vi "LEDS.vi"(7 "Action":T1, 8 "error in":errorcluster, 10 "On/Off":bool) -> (0 "error out":errorcluster)   [LabVIEW 2013]
uses:
  LEDSaction.ctl
  <vilib>/Rock Robotics/SystemInterfaces/DIO/FPGA_DIOChannel.ctl
  <vilib>/Rock Robotics/SystemInterfaces/Typedef/FPGA_TypedefDigitalModule.ctl
panel:
  out "PressureHigh":bool
  out "PressureLow":bool
  out "Shoot":bool
  out "Shift":bool
  out "Hot":bool
  out "NotHot":bool
  out "10 Seconds":bool
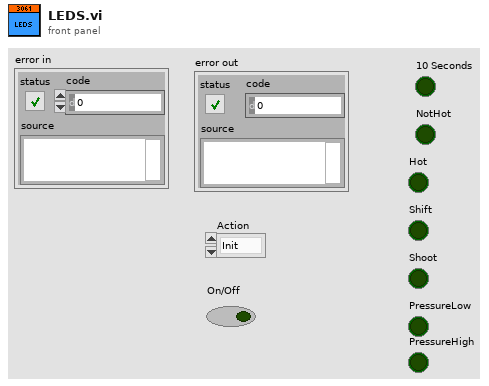
[diagram p1: front panel]
types:
  T1 = typedef "LEDSaction.ctl" = enum16{"Init", "10SecondsLeft", "LimitDown", "LimitUp", "CollectDown", "CollectUp", "NotHot", "Hot", "Shift", "RollBack", "RollFwd", "Shoot", "Distance Low", "DistanceHigh", "PressureLow", "PressureHigh"}
  T2 = typedef "FPGA_DIOChannel.ctl" = enum8{"DIO 1", "DIO 2", "DIO 3", "DIO 4", "DIO 5", "DIO 6", "DIO 7", "DIO 8", "DIO 9", "DIO 10", "DIO 11", "DIO 12", "DIO 13", "DIO 14", "Invalid"}
  T3 = typedef "FPGA_TypedefDigitalModule.ctl" = enum16{"Digital Module 1", "Digital Module 2"}
  T4 = typedef "WPI_DigitalOutputDevRef.ctl" = cluster{"Digital Module":T3, "DIO Channel":T2, "DevStatus":errorcluster}
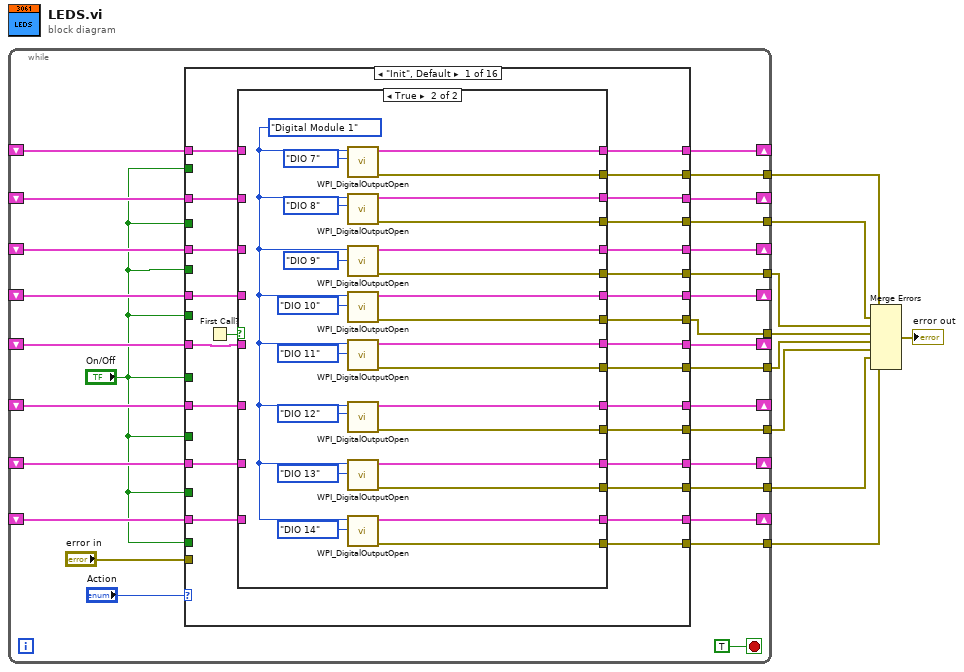
[diagram p0: block diagram]
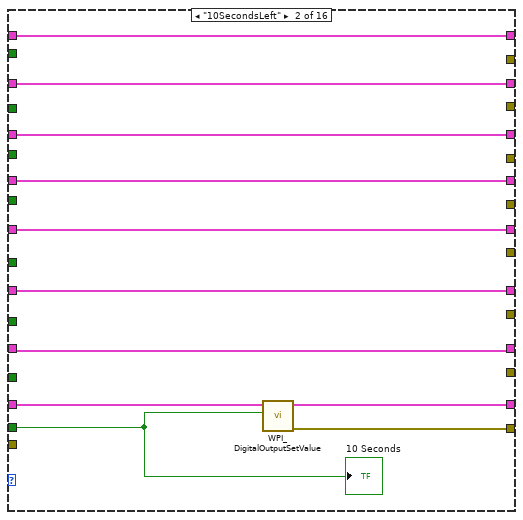
[diagram p3: hidden frame]
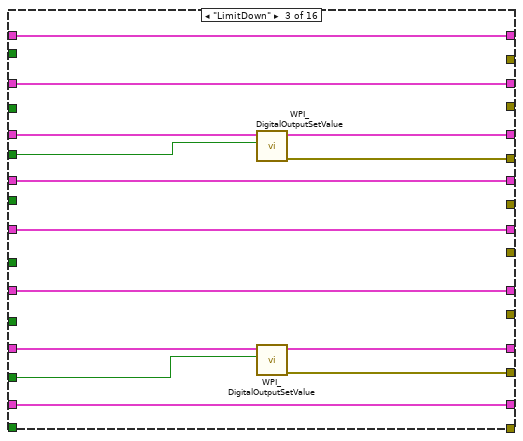
[diagram p4: hidden frame]
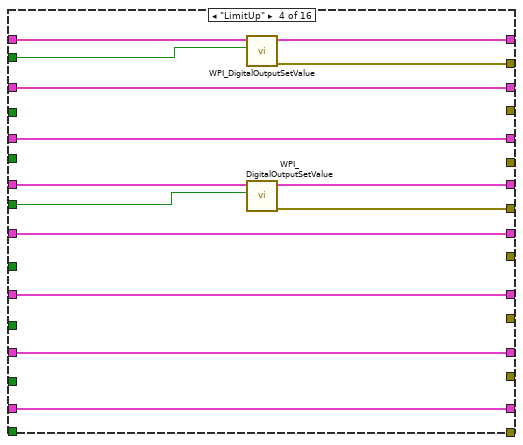
[diagram p5: hidden frame]
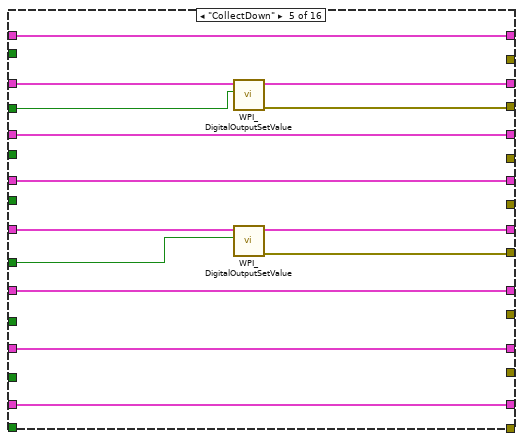
[diagram p6: hidden frame]
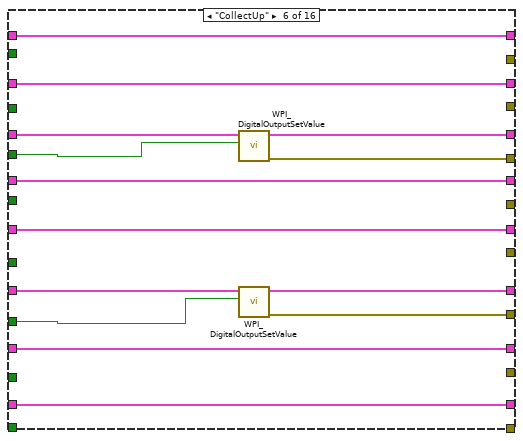
[diagram p7: hidden frame]
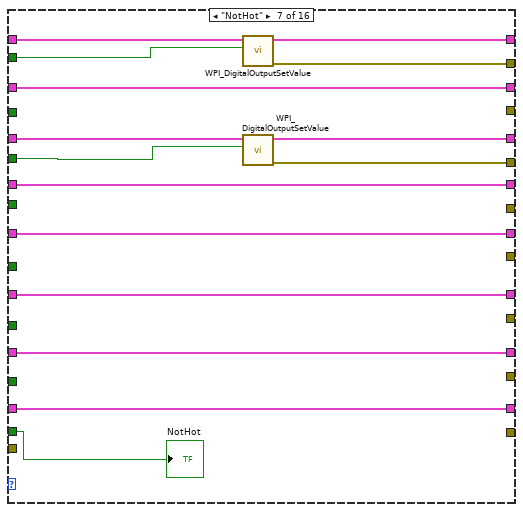
[diagram p8: hidden frame]
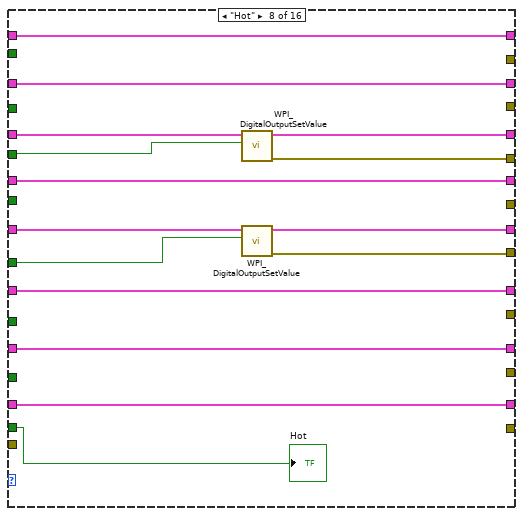
[diagram p9: hidden frame]
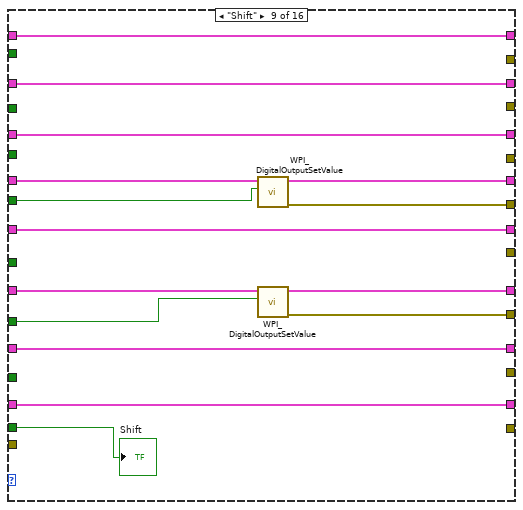
[diagram p10: hidden frame]
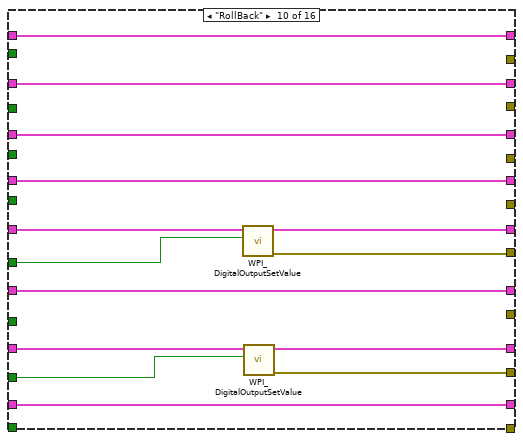
[diagram p11: hidden frame]
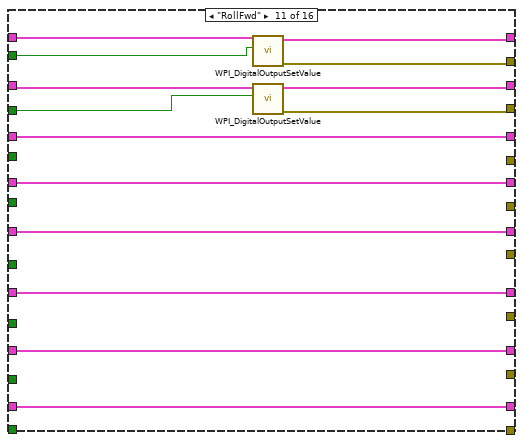
[diagram p12: hidden frame]
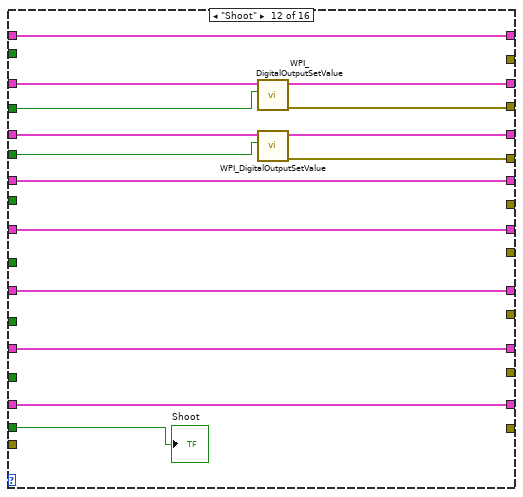
[diagram p13: hidden frame]
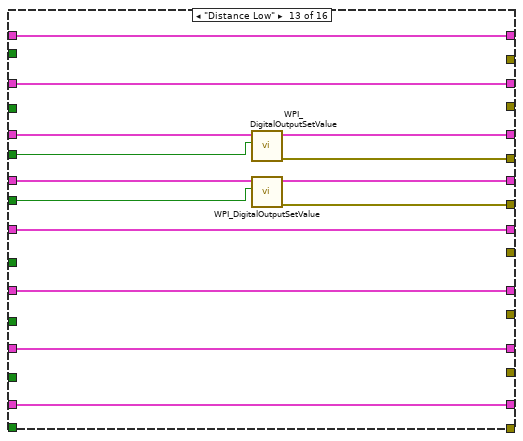
[diagram p14: hidden frame]
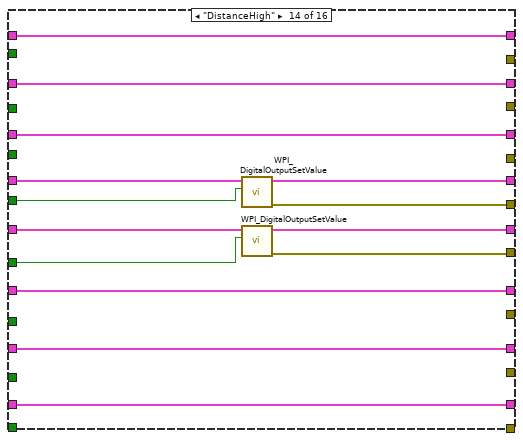
[diagram p15: hidden frame]
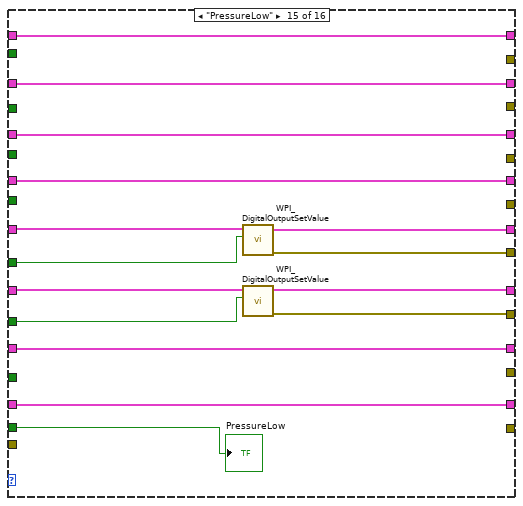
[diagram p16: hidden frame]
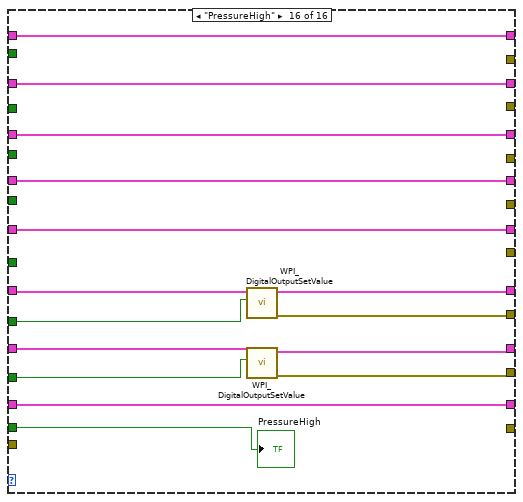
[diagram p17: hidden frame]
diagram:
  n1 = while {
    shift-right: [w37] -> _
    shift-left: _ -> [w29]
    shift-right: [w36] -> _
    shift-left: _ -> [w28]
    shift-right: [w35] -> _
    shift-left: _ -> [w27]
    shift-right: [w34] -> _
    shift-left: _ -> [w26]
    shift-right: [w33] -> _
    shift-left: _ -> [w25]
    shift-right: [w32] -> _
    shift-left: _ -> [w24]
    shift-right: [w31] -> _
    shift-left: _ -> [w23]
    shift-right: [w30] -> _
    shift-left: _ -> [w22]
    tunnel: [w20] -> w8
    tunnel: [w19] -> w7
    tunnel: [w18] -> w6
    tunnel: [w17] -> w5
    tunnel: [w16] -> w4
    tunnel: [w15] -> w3
    tunnel: [w14] -> w2
    tunnel: [w13] -> w1
    stop <- TRUE stop-if-true
    n2 = case shown="\"Init\", Default" "Action" {
      tunnel: [w47 w104 w111 w134 w144 w158 w176 w186 w200 w212 w235 w246 w260 w272 w284 w299] -> w37
      tunnel: [w49 w103 w112 w129 w148 w157 w173 w187 w201 w213 w234 w250 w259 w273 w285 w300] -> w36
      tunnel: [w51 w102 w119 w130 w143 w162 w177 w192 w202 w214 w231 w249 w264 w274 w286 w301] -> w35
      tunnel: [w53 w101 w113 w133 w142 w156 w172 w188 w206 w215 w230 w245 w263 w277 w287 w302] -> w34
      tunnel: [w55 w100 w114 w128 w147 w155 w171 w191 w203 w220 w229 w244 w258 w278 w292 w303] -> w33
      tunnel: [w57 w99 w115 w127 w141 w161 w170 w185 w207 w217 w228 w243 w257 w271 w293 w307] -> w32
      tunnel: [w59 w98 w118 w126 w140 w154 w169 w184 w199 w221 w227 w242 w256 w270 w289 w308] -> w31
      tunnel: [w61 w105 w116 w125 w139 w153 w168 w183 w198 w216 w226 w241 w255 w269 w288 w304] -> w30
      tunnel: w29 -> [w38 w104 w111 w132 w144 w158 w175 w186 w200 w212 w232 w246 w260 w272 w284 w299]
      tunnel: w28 -> [w39 w103 w112 w129 w145 w157 w173 w187 w201 w213 w233 w247 w259 w273 w285 w300]
      tunnel: w27 -> [w40 w102 w120 w130 w143 w159 w174 w190 w202 w214 w231 w248 w261 w274 w286 w301]
      tunnel: w26 -> [w41 w101 w113 w131 w142 w156 w172 w188 w205 w215 w230 w245 w262 w276 w287 w302]
      tunnel: w25 -> [w45 w100 w114 w128 w146 w155 w171 w189 w203 w218 w229 w244 w258 w275 w291 w303]
      tunnel: w24 -> [w44 w99 w115 w127 w141 w160 w170 w185 w204 w217 w228 w243 w257 w271 w290 w306]
      tunnel: w23 -> [w43 w98 w117 w126 w140 w154 w169 w184 w199 w219 w227 w242 w256 w270 w289 w305]
      tunnel: w22 -> [w42 w106 w116 w125 w139 w153 w168 w183 w198 w216 w226 w241 w255 w269 w288 w304]
      tunnel: [w48 _ _ w124 _ _ w167 _ _ _ w225 _ _ _ _ _] -> w13
      tunnel: [w50 _ _ _ w138 _ _ _ _ _ w224 w240 _ _ _ _] -> w14
      tunnel: [w52 _ w110 _ _ w152 w166 w182 _ _ _ w239 w254 _ _ _] -> w15
      tunnel: [w54 _ _ w123 _ _ _ _ w197 _ _ _ w253 w268 _ _] -> w16
      tunnel: [w56 _ _ _ w137 _ _ w181 _ w211 _ _ _ w267 w283 _] -> w17
      tunnel: [w58 _ _ _ _ w151 _ _ w196 _ _ _ _ _ w282 w298] -> w18
      tunnel: [w60 _ w109 _ _ _ _ _ _ w210 _ _ _ _ _ w297] -> w19
      tunnel: [w62 w97 _ _ _ _ _ _ _ _ _ _ _ _ _ _] -> w20
      tunnel: "On/Off" -> [_ _ _ _ w135 _ _ w179 _ w209 _ _ _ w265 w281 _]
      tunnel: "On/Off" -> [_ _ _ w122 _ _ w165 _ _ _ w222 _ _ _ _ _]
      tunnel: "On/Off" -> [_ _ _ _ w136 _ _ _ _ _ w223 w238 _ _ _ _]
      tunnel: "On/Off" -> [_ _ w107 _ _ w150 w164 w180 _ _ _ w237 w252 _ _ _]
      tunnel: "On/Off" -> [_ _ _ w121 _ _ _ _ w195 _ _ _ w251 w266 _ _]
      tunnel: "On/Off" -> [_ w96 _ _ _ _ w163 w178 w193 _ _ w236 _ _ w279 w294]
      tunnel: "On/Off" -> [_ _ w108 _ _ _ _ _ _ w208 _ _ _ _ _ w295]
      tunnel: "On/Off" -> [_ _ _ _ _ w149 _ _ w194 _ _ _ _ _ w280 w296]
      tunnel: "error in" -> [_ _ _ _ _ _ _ _ _ _ _ _ _ _ _ _]
      frame "Init", Default {
        n3 = First Call?() -> (First Call?: T/F=w46:bool)
        n4 = case shown="True" w46 {
          tunnel: [_ w87] -> w62
          tunnel: [w67 w86] -> w61
          tunnel: [_ w85] -> w60
          tunnel: [w68 w84] -> w59
          tunnel: [_ w83] -> w58
          tunnel: [w69 w82] -> w57
          tunnel: [_ w81] -> w56
          tunnel: [w70 w80] -> w55
          tunnel: [_ w79] -> w54
          tunnel: [w66 w78] -> w53
          tunnel: [_ w77] -> w52
          tunnel: [w65 w76] -> w51
          tunnel: [_ w75] -> w50
          tunnel: [w64 w74] -> w49
          tunnel: [_ w73] -> w48
          tunnel: [w63 w72] -> w47
          tunnel: w45 -> [w70 _]
          tunnel: w44 -> [w69 _]
          tunnel: w43 -> [w68 _]
          tunnel: w42 -> [w67 _]
          tunnel: w41 -> [w66 _]
          tunnel: w40 -> [w65 _]
          tunnel: w39 -> [w64 _]
          tunnel: w38 -> [w63 _]
          frame False {
          }
          frame True {
            w71 = FPGA_TypedefDigitalModule."Digital Module 1" ("Digital Module (Module 1)")
            n5 = call <vilib>:"WPI_DigitalOutputOpen.vi"("DIO Channel"=FPGA_DIOChannel."DIO 7", "Digital Module (Module 1)"=w71) -> ("error out"=w73:errorcluster, "DigitalOutputDevRef"=w72:T4)  [unwired: 8 in]
            n6 = call <vilib>:"WPI_DigitalOutputOpen.vi"("DIO Channel"=FPGA_DIOChannel."DIO 8", "Digital Module (Module 1)"=w71) -> ("error out"=w75:errorcluster, "DigitalOutputDevRef"=w74:T4)  [unwired: 8 in]
            n7 = call <vilib>:"WPI_DigitalOutputOpen.vi"("DIO Channel"=FPGA_DIOChannel."DIO 9", "Digital Module (Module 1)"=w71) -> ("error out"=w77:errorcluster, "DigitalOutputDevRef"=w76:T4)  [unwired: 8 in]
            n8 = call <vilib>:"WPI_DigitalOutputOpen.vi"("DIO Channel"=FPGA_DIOChannel."DIO 10", "Digital Module (Module 1)"=w71) -> ("error out"=w79:errorcluster, "DigitalOutputDevRef"=w78:T4)  [unwired: 8 in]
            n9 = call <vilib>:"WPI_DigitalOutputOpen.vi"("DIO Channel"=FPGA_DIOChannel."DIO 11", "Digital Module (Module 1)"=w71) -> ("error out"=w81:errorcluster, "DigitalOutputDevRef"=w80:T4)  [unwired: 8 in]
            n10 = call <vilib>:"WPI_DigitalOutputOpen.vi"("DIO Channel"=FPGA_DIOChannel."DIO 12", "Digital Module (Module 1)"=w71) -> ("error out"=w83:errorcluster, "DigitalOutputDevRef"=w82:T4)  [unwired: 8 in]
            n11 = call <vilib>:"WPI_DigitalOutputOpen.vi"("DIO Channel"=FPGA_DIOChannel."DIO 13", "Digital Module (Module 1)"=w71) -> ("error out"=w85:errorcluster, "DigitalOutputDevRef"=w84:T4)  [unwired: 8 in]
            n12 = call <vilib>:"WPI_DigitalOutputOpen.vi"("DIO Channel"=FPGA_DIOChannel."DIO 14", "Digital Module (Module 1)"=w71) -> ("error out"=w87:errorcluster, "DigitalOutputDevRef"=w86:T4)  [unwired: 8 in]
          }
        }
      }
      frame "10SecondsLeft" {
        n13 = call <vilib>:"WPI_DigitalOutputSetValue.vi"("Value"=w96, "DigitalOutputDevRef"=w106) -> ("error out"=w97:errorcluster, "DigitalOutputDevRef"=w105:T4)  [unwired: 8 in]
        "10 Seconds" <- w96
      }
      frame "LimitDown" {
        n14 = call <vilib>:"WPI_DigitalOutputSetValue.vi"("Value"=w107, "DigitalOutputDevRef"=w120) -> ("error out"=w110:errorcluster, "DigitalOutputDevRef"=w119:T4)  [unwired: 8 in]
        n15 = call <vilib>:"WPI_DigitalOutputSetValue.vi"("Value"=w108, "DigitalOutputDevRef"=w117) -> ("error out"=w109:errorcluster, "DigitalOutputDevRef"=w118:T4)  [unwired: 8 in]
      }
      frame "LimitUp" {
        n16 = call <vilib>:"WPI_DigitalOutputSetValue.vi"("Value"=w122, "DigitalOutputDevRef"=w132) -> ("error out"=w124:errorcluster, "DigitalOutputDevRef"=w134:T4)  [unwired: 8 in]
        n17 = call <vilib>:"WPI_DigitalOutputSetValue.vi"("Value"=w121, "DigitalOutputDevRef"=w131) -> ("error out"=w123:errorcluster, "DigitalOutputDevRef"=w133:T4)  [unwired: 8 in]
      }
      frame "CollectDown" {
        n18 = call <vilib>:"WPI_DigitalOutputSetValue.vi"("Value"=w136, "DigitalOutputDevRef"=w145) -> ("error out"=w138:errorcluster, "DigitalOutputDevRef"=w148:T4)  [unwired: 8 in]
        n19 = call <vilib>:"WPI_DigitalOutputSetValue.vi"("Value"=w135, "DigitalOutputDevRef"=w146) -> ("error out"=w137:errorcluster, "DigitalOutputDevRef"=w147:T4)  [unwired: 8 in]
      }
      frame "CollectUp" {
        n20 = call <vilib>:"WPI_DigitalOutputSetValue.vi"("Value"=w150, "DigitalOutputDevRef"=w159) -> ("error out"=w152:errorcluster, "DigitalOutputDevRef"=w162:T4)  [unwired: 8 in]
        n21 = call <vilib>:"WPI_DigitalOutputSetValue.vi"("Value"=w149, "DigitalOutputDevRef"=w160) -> ("error out"=w151:errorcluster, "DigitalOutputDevRef"=w161:T4)  [unwired: 8 in]
      }
      frame "NotHot" {
        n22 = call <vilib>:"WPI_DigitalOutputSetValue.vi"("Value"=w165, "DigitalOutputDevRef"=w175) -> ("error out"=w167:errorcluster, "DigitalOutputDevRef"=w176:T4)  [unwired: 8 in]
        n23 = call <vilib>:"WPI_DigitalOutputSetValue.vi"("Value"=w164, "DigitalOutputDevRef"=w174) -> ("error out"=w166:errorcluster, "DigitalOutputDevRef"=w177:T4)  [unwired: 8 in]
        "NotHot" <- w163
      }
      frame "Hot" {
        n24 = call <vilib>:"WPI_DigitalOutputSetValue.vi"("Value"=w180, "DigitalOutputDevRef"=w190) -> ("error out"=w182:errorcluster, "DigitalOutputDevRef"=w192:T4)  [unwired: 8 in]
        n25 = call <vilib>:"WPI_DigitalOutputSetValue.vi"("Value"=w179, "DigitalOutputDevRef"=w189) -> ("error out"=w181:errorcluster, "DigitalOutputDevRef"=w191:T4)  [unwired: 8 in]
        "Hot" <- w178
      }
      frame "Shift" {
        n26 = call <vilib>:"WPI_DigitalOutputSetValue.vi"("Value"=w195, "DigitalOutputDevRef"=w205) -> ("error out"=w197:errorcluster, "DigitalOutputDevRef"=w206:T4)  [unwired: 8 in]
        n27 = call <vilib>:"WPI_DigitalOutputSetValue.vi"("Value"=w194, "DigitalOutputDevRef"=w204) -> ("error out"=w196:errorcluster, "DigitalOutputDevRef"=w207:T4)  [unwired: 8 in]
        "Shift" <- w193
      }
      frame "RollBack" {
        n28 = call <vilib>:"WPI_DigitalOutputSetValue.vi"("Value"=w209, "DigitalOutputDevRef"=w218) -> ("error out"=w211:errorcluster, "DigitalOutputDevRef"=w220:T4)  [unwired: 8 in]
        n29 = call <vilib>:"WPI_DigitalOutputSetValue.vi"("Value"=w208, "DigitalOutputDevRef"=w219) -> ("error out"=w210:errorcluster, "DigitalOutputDevRef"=w221:T4)  [unwired: 8 in]
      }
      frame "RollFwd" {
        n30 = call <vilib>:"WPI_DigitalOutputSetValue.vi"("Value"=w222, "DigitalOutputDevRef"=w232) -> ("error out"=w225:errorcluster, "DigitalOutputDevRef"=w235:T4)  [unwired: 8 in]
        n31 = call <vilib>:"WPI_DigitalOutputSetValue.vi"("Value"=w223, "DigitalOutputDevRef"=w233) -> ("error out"=w224:errorcluster, "DigitalOutputDevRef"=w234:T4)  [unwired: 8 in]
      }
      frame "Shoot" {
        n32 = call <vilib>:"WPI_DigitalOutputSetValue.vi"("Value"=w238, "DigitalOutputDevRef"=w247) -> ("error out"=w240:errorcluster, "DigitalOutputDevRef"=w250:T4)  [unwired: 8 in]
        n33 = call <vilib>:"WPI_DigitalOutputSetValue.vi"("Value"=w237, "DigitalOutputDevRef"=w248) -> ("error out"=w239:errorcluster, "DigitalOutputDevRef"=w249:T4)  [unwired: 8 in]
        "Shoot" <- w236
      }
      frame "Distance Low" {
        n34 = call <vilib>:"WPI_DigitalOutputSetValue.vi"("Value"=w252, "DigitalOutputDevRef"=w261) -> ("error out"=w254:errorcluster, "DigitalOutputDevRef"=w264:T4)  [unwired: 8 in]
        n35 = call <vilib>:"WPI_DigitalOutputSetValue.vi"("Value"=w251, "DigitalOutputDevRef"=w262) -> ("error out"=w253:errorcluster, "DigitalOutputDevRef"=w263:T4)  [unwired: 8 in]
      }
      frame "DistanceHigh" {
        n36 = call <vilib>:"WPI_DigitalOutputSetValue.vi"("Value"=w266, "DigitalOutputDevRef"=w276) -> ("error out"=w268:errorcluster, "DigitalOutputDevRef"=w277:T4)  [unwired: 8 in]
        n37 = call <vilib>:"WPI_DigitalOutputSetValue.vi"("Value"=w265, "DigitalOutputDevRef"=w275) -> ("error out"=w267:errorcluster, "DigitalOutputDevRef"=w278:T4)  [unwired: 8 in]
      }
      frame "PressureLow" {
        n38 = call <vilib>:"WPI_DigitalOutputSetValue.vi"("Value"=w281, "DigitalOutputDevRef"=w291) -> ("error out"=w283:errorcluster, "DigitalOutputDevRef"=w292:T4)  [unwired: 8 in]
        n39 = call <vilib>:"WPI_DigitalOutputSetValue.vi"("Value"=w280, "DigitalOutputDevRef"=w290) -> ("error out"=w282:errorcluster, "DigitalOutputDevRef"=w293:T4)  [unwired: 8 in]
        "PressureLow" <- w279
      }
      frame "PressureHigh" {
        n40 = call <vilib>:"WPI_DigitalOutputSetValue.vi"("Value"=w296, "DigitalOutputDevRef"=w306) -> ("error out"=w298:errorcluster, "DigitalOutputDevRef"=w307:T4)  [unwired: 8 in]
        n41 = call <vilib>:"WPI_DigitalOutputSetValue.vi"("Value"=w295, "DigitalOutputDevRef"=w305) -> ("error out"=w297:errorcluster, "DigitalOutputDevRef"=w308:T4)  [unwired: 8 in]
        "PressureHigh" <- w294
      }
    }
  }
  n42 = Merge Errors(w1, w2, w3, w4, w5, w6, w7, w8) -> (→"error out":errorcluster)
